vi "梦幻城堡C6~20通信.vi"() -> ()   [LabVIEW 2016, in "环境动力监测库.lvlib"]
uses:
  <vilib>/Instr/_visa.llb/VISA Configure Serial Port (Instr).vi
panel:
  in  "open":bool
  in  "close":bool
  in  "串口重开":bool
  in  "timeout (10sec)":u32=10000 caption="超时（10秒）"
  out "通信指示":bool
  in  "关机":bool
  in  "功率查询":bool
  in  "状态查询":bool
  in  "写入缓冲区":string
  out "读取缓冲区":string
  in  "stop bits (10: 1 bit)":u16(ring)=10 caption="停止位（10: 1位）" items=["1.0"=10, "1.5"=15, "2.0"=20]
  in  "parity (0:none)":enum16{"None", "Odd", "Even", "Mark", "Space"}(ring) caption="奇偶（0:无）"
  in  "data bits (8)":u16=8 caption="数据比特(8)" min=5 max=8 step=1
  in  "baud rate (9600)":u32=9600 caption="波特率(9600)"
  in  "VISA resource name":refnum<visa-resource-name> caption="VISA资源名称"
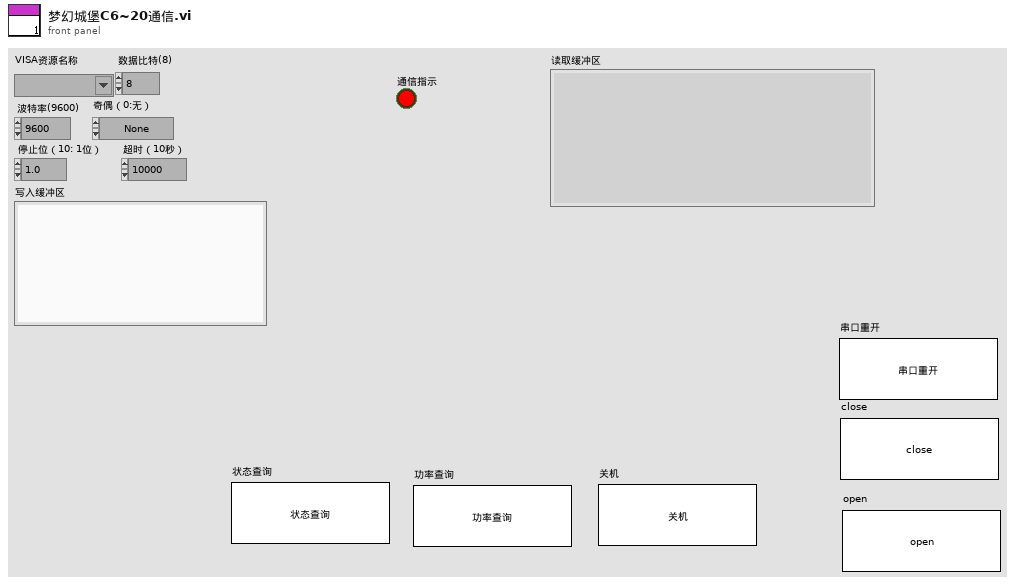
[diagram p1: front panel]
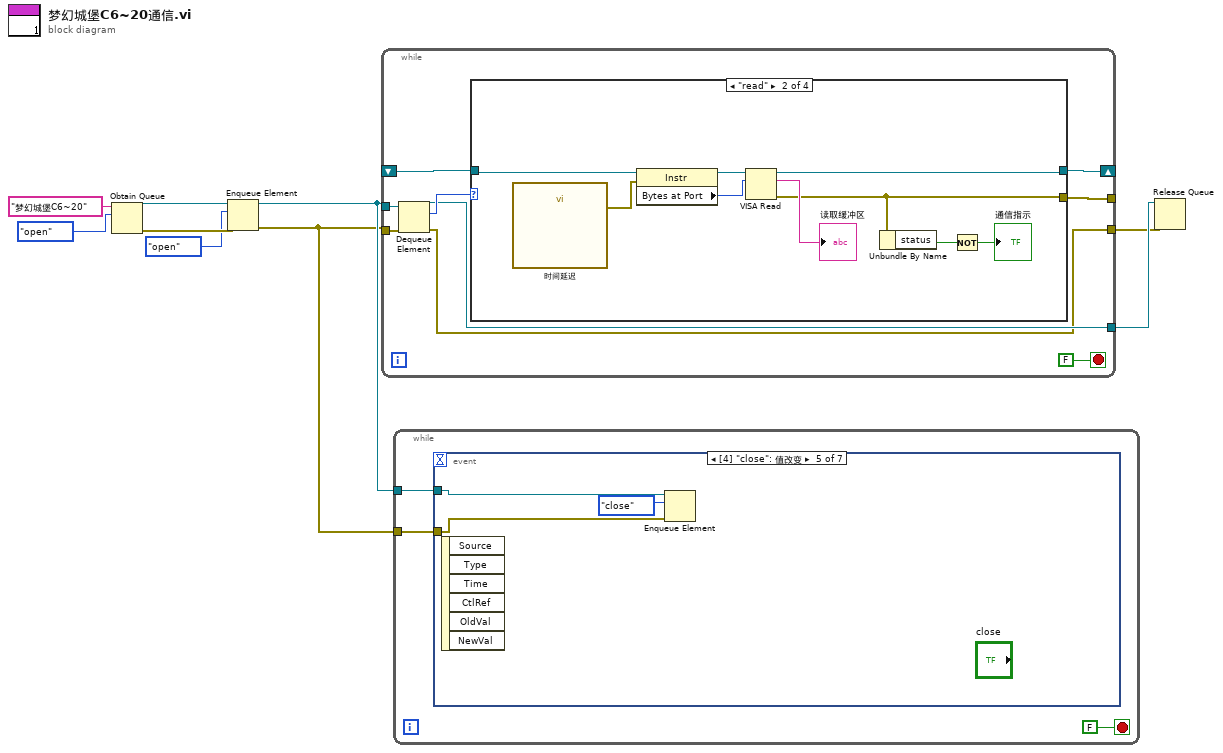
[diagram p0: block diagram]
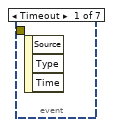
[diagram p2: hidden frame]
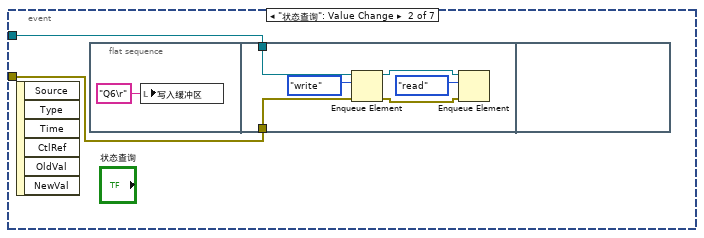
[diagram p3: hidden frame]
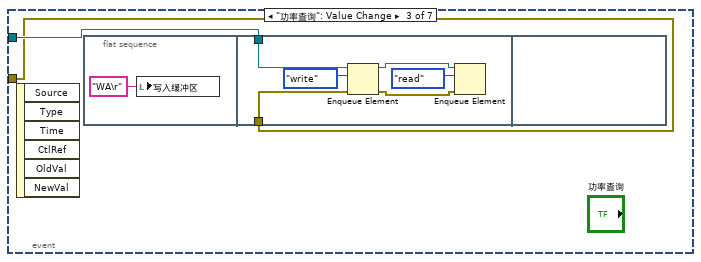
[diagram p4: hidden frame]
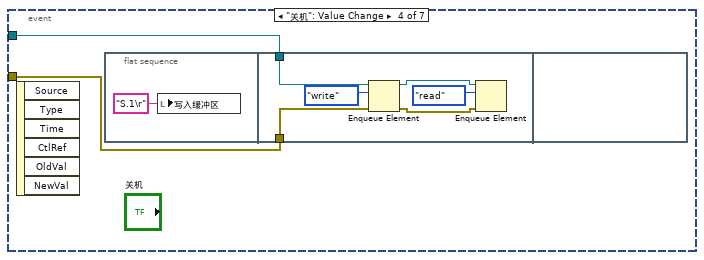
[diagram p5: hidden frame]
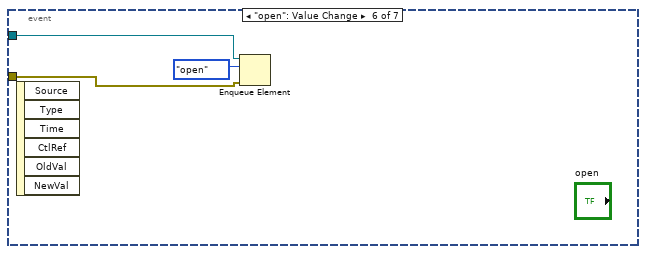
[diagram p6: hidden frame]
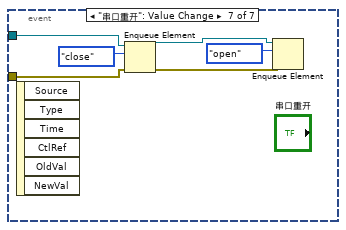
[diagram p7: hidden frame]
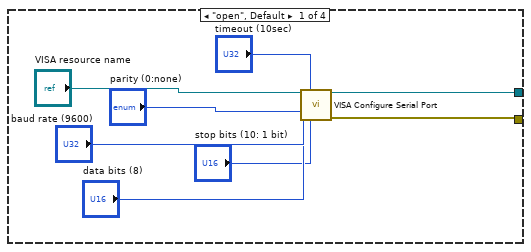
[diagram p8: hidden frame]
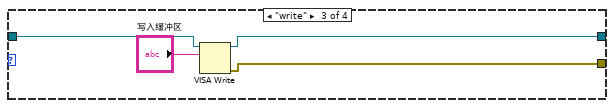
[diagram p9: hidden frame]
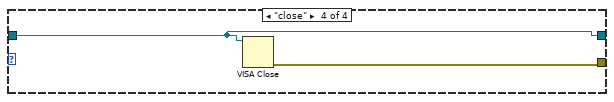
[diagram p10: hidden frame]
diagram:
  n1 = Obtain Queue(name (unnamed)="梦幻城堡C6~20" ("名称（未命名）"), element data type=enum16{"open", "read", "write", "close"}."open") -> (queue out=w5:refnum<queue>, error out=w4:errorcluster)  [unwired: 3 in, 1 out]
  n2 = Enqueue Element(queue=w5, element=enum16{"open", "read", "write", "close"}."open", error in (no error)=w4) -> (queue out=w2:refnum<queue>, error out=w1:errorcluster)  [unwired: 1 in, 1 out]
  n3 = while {
    shift-right: [w18] -> _
    shift-left: _ -> [w17]
    tunnel: [w16] -> _
    tunnel: w2 -> [w14]
    tunnel: w1 -> [w13]
    tunnel: [w11] -> w7
    tunnel: [w10] -> w6
    stop <- FALSE stop-if-true
    n4 = Dequeue Element(queue=w14, error in (no error)=w13) -> (queue out=w11:refnum<queue>, element=w12:enum16{"open", "read", "write", "close"}, error out=w10:errorcluster)  [unwired: 1 in, 1 out]
    n5 = case shown="\"read\"" w12 {
      tunnel: [w21 w32 w37 w40] -> w18
      tunnel: w17 -> [_ w35 w39 w40]
      tunnel: [w20 w30 w36 w41] -> w16
      frame "open", Default {
        n6 = call-poly "VISA Configure Serial Port"("VISA resource name"="VISA resource name", "timeout (10sec)"="timeout (10sec)", "baud rate (9600)"="baud rate (9600)", "data bits (8)"="data bits (8)", "parity (0:none)"="parity (0:none)", "stop bits (10: 1 bit)"="stop bits (10: 1 bit)") -> ("VISA resource name out"=w21:refnum<visa-resource-name>, "error out"=w20:errorcluster)  [unwired: 8 in]
      }
      frame "read" {
        n7 = call "时间延迟"() -> ("error out"=w27:errorcluster)  [unwired: 11 in]
        n8 = property class="Instr"(reference=w35, error in=w27) -> (reference out=w33:refnum<visa-resource-name>, "Bytes at Port"=w34:u32)  [unwired: 1 out]
        n9 = VISA Read(VISA resource name=w33, byte count=w34) -> (VISA resource name out=w32:refnum<visa-resource-name>, read buffer=→"读取缓冲区":string, error out=w30:errorcluster)  [unwired: 1 in, 1 out]
        n10 = Unbundle By Name(w30) -> ("status"=w29:bool)
        n11 = Not(x=w29) -> (.not. x?=→"通信指示":bool)
      }
      frame "write" {
        n12 = VISA Write(VISA resource name=w39, write buffer="写入缓冲区") -> (VISA resource name out=w37:refnum<visa-resource-name>, error out=w36:errorcluster)  [unwired: 1 in, 1 out]
      }
      frame "close" {
        n13 = VISA Close(VISA resource name=w40) -> (error out=w41:errorcluster)  [unwired: 1 in]
      }
    }
  }
  n14 = while {
    tunnel: w2 -> [w43]
    tunnel: w1 -> [w42]
    stop <- FALSE stop-if-true
    n15 = event shown="[4] \"close\": 值改变" {
      selector: _ -> [_ _ _ _ _ _ _]
      dyn-events: _ -> [_ _ _ _ _ _ _]
      timeout: _ -> [_ _ _ _ _ _ _]
      tunnel: w43 -> [_ w46 w55 w64 w74 w76 w81]
      tunnel: w42 -> [_ w45 w54 w63 w73 w75 w80]
      event Timeout {
        n16 = event-data() -> ()  [unwired: 1 in, 3 out]
      }
      event "状态查询": Value Change {
        n17 = event-data() -> ()  [unwired: 1 in, 6 out]
        n18 = flat-sequence {
          tunnel: w46 -> [w53]
          tunnel: w45 -> [w52]
          frame #0 {
            n19 = local write "写入缓冲区"("Q6\r" ("写入缓冲区")) -> ()
          }
          frame #1 {
            n20 = Enqueue Element(queue=w53, element=enum16{"open", "read", "write", "close"}."write" ("元素"), error in (no error)=w52) -> (queue out=w50:refnum<queue>, error out=w49:errorcluster)  [unwired: 1 in, 1 out]
            n21 = Enqueue Element(queue=w50, element=enum16{"open", "read", "write", "close"}."read" ("元素"), error in (no error)=w49) -> ()  [unwired: 1 in, 3 out]
          }
          frame #2 {
          }
        }
      }
      event "功率查询": Value Change {
        n22 = event-data() -> ()  [unwired: 1 in, 6 out]
        n23 = flat-sequence {
          tunnel: w55 -> [w62]
          tunnel: w54 -> [w61]
          frame #0 {
            n24 = local write "写入缓冲区"("WA\r" ("写入缓冲区")) -> ()
          }
          frame #1 {
            n25 = Enqueue Element(queue=w62, element=enum16{"open", "read", "write", "close"}."write" ("元素"), error in (no error)=w61) -> (queue out=w59:refnum<queue>, error out=w58:errorcluster)  [unwired: 1 in, 1 out]
            n26 = Enqueue Element(queue=w59, element=enum16{"open", "read", "write", "close"}."read" ("元素"), error in (no error)=w58) -> ()  [unwired: 1 in, 3 out]
          }
          frame #2 {
          }
        }
      }
      event "关机": Value Change {
        n27 = event-data() -> ()  [unwired: 1 in, 6 out]
        n28 = flat-sequence {
          tunnel: w64 -> [w71]
          tunnel: w63 -> [w70]
          frame #0 {
            n29 = local write "写入缓冲区"("S.1\r" ("写入缓冲区")) -> ()
          }
          frame #1 {
            n30 = Enqueue Element(queue=w71, element=enum16{"open", "read", "write", "close"}."write" ("元素"), error in (no error)=w70) -> (queue out=w68:refnum<queue>, error out=w67:errorcluster)  [unwired: 1 in, 1 out]
            n31 = Enqueue Element(queue=w68, element=enum16{"open", "read", "write", "close"}."read" ("元素"), error in (no error)=w67) -> ()  [unwired: 1 in, 3 out]
          }
          frame #2 {
          }
        }
      }
      event "close": Value Change {
        n32 = event-data() -> ()  [unwired: 1 in, 6 out]
        n33 = Enqueue Element(queue=w74, element=enum16{"open", "read", "write", "close"}."close" ("元素"), error in (no error)=w73) -> ()  [unwired: 1 in, 3 out]
      }
      event "open": Value Change {
        n34 = event-data() -> ()  [unwired: 1 in, 6 out]
        n35 = Enqueue Element(queue=w76, element=enum16{"open", "read", "write", "close"}."open" ("元素"), error in (no error)=w75) -> ()  [unwired: 1 in, 3 out]
      }
      event "串口重开": Value Change {
        n36 = event-data() -> ()  [unwired: 1 in, 6 out]
        n37 = Enqueue Element(queue=w81, element=enum16{"open", "read", "write", "close"}."close" ("元素"), error in (no error)=w80) -> (queue out=w79:refnum<queue>, error out=w78:errorcluster)  [unwired: 1 in, 1 out]
        n38 = Enqueue Element(queue=w79, element=enum16{"open", "read", "write", "close"}."open" ("元素"), error in (no error)=w78) -> ()  [unwired: 1 in, 3 out]
      }
    }
  }
  n39 = Release Queue(queue=w7, error in (no error)=w6) -> ()  [unwired: 1 in, 3 out]
